vi "Calibrate LCVR_Capture.vi"(8 "error in (no error)":errorcluster {"code" format="%.0x"}, 10 "Handle in":u32, 11 "Buffer Info":T1) -> (0 "error out":errorcluster, 1 "Image":dbl[][](graph), 2 "Handle out":u32, 3 "contrast":dbl)   [LabVIEW 2012]
panel:
  out "frame":i32
  out "Frame Count":i32
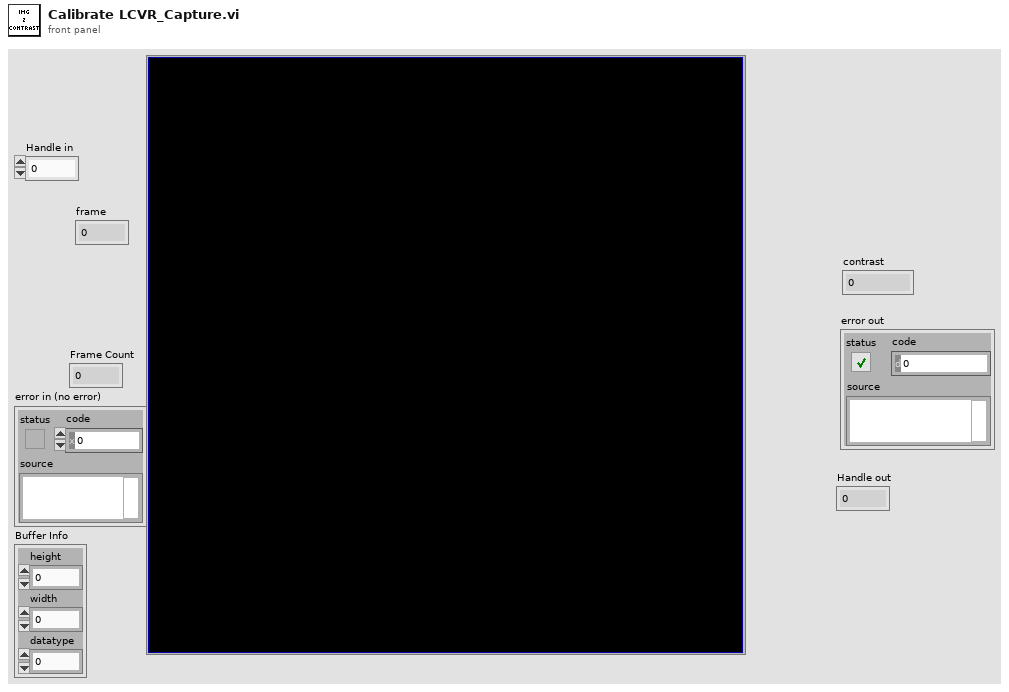
[diagram p1: front panel]
types:
  T1 = cluster{"height":u32, "width":u32, "datatype":u32}
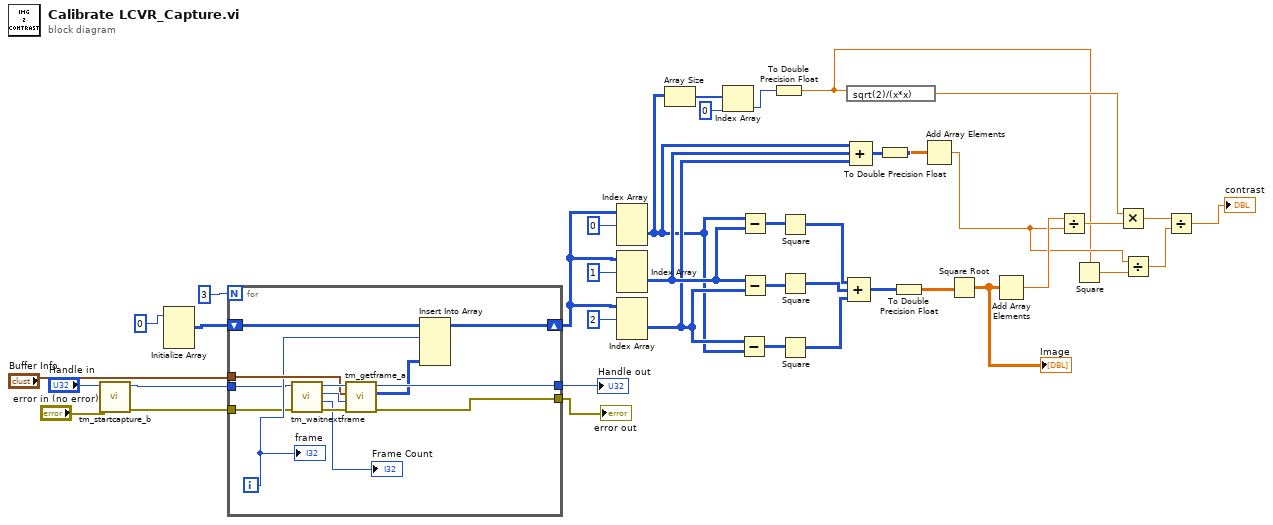
[diagram p0: block diagram]
diagram:
  n1 = call <userlib>:"tm_startcapture_b.vi"("error in (no error)"="error in (no error)", "Handle in"="Handle in") -> ("error out"=w36:errorcluster, "Handle out"=w37:u32)  [unwired: 8 in]
  n2 = Initialize Array(u16 0 ("element")) -> (w39:u16[][][])  [unwired: 3 in]
  n3 = for {
    N: 3 -> [_]
    tunnel: "Buffer Info" -> [w50]
    tunnel: [w49] -> w32
    tunnel: [w48] -> w31
    shift-right: [w46] -> w30
    shift-left: w39 -> [w47]
    tunnel: w37 -> [w43]
    tunnel: w36 -> [w42]
    i -> [w45]
    n4 = call <userlib>:"tm_waitnextframe.vi"("error in (no error)"=w42, "Handle in"=w43) -> ("error out"=w51:errorcluster, "Frame Count"=→"Frame Count":i32, "Frame Index"=w53:i32, "Handle out"=w52:u32)  [unwired: 6 in]
    n5 = call <userlib>:"tm_getframe_a.vi"("error in (no error)"=w51, "Frame Index"=w53, "Buffer Info"=w50, "Handle in"=w52) -> ("error out"=w48:errorcluster, "Data 16"=w41:u16[][], "Handle out"=w49:u32)  [unwired: 3 in, 2 out]
    n6 = Insert Into Array(array=w47, index (dim 0)=w45, new element=w41) -> (w46:u16[][][])  [unwired: 2 in]
    "frame" <- w45
  }
  "Handle out" <- w32
  "error out" <- w31
  n7 = Index Array(array=w30, index (dim 0)=0 ("index (page)")) -> (element=w16:u16[][])  [unwired: 2 in]
  n8 = Index Array(array=w30, index (dim 0)=1 ("index (page)")) -> (element=w19:u16[][])  [unwired: 2 in]
  n9 = Index Array(array=w30, index (dim 0)=2 ("index (page)")) -> (element=w18:u16[][])  [unwired: 2 in]
  n10 = Array Size(array=w16) -> (size(s)=w15:i32[])
  n11 = Index Array(array=w15, index=0) -> (element=w10:i32)
  n12 = Subtract(x=w18, y=w16) -> (x-y=w24:u16[][])
  n13 = Subtract(x=w16, y=w19) -> (x-y=w26:u16[][])
  n14 = Subtract(x=w19, y=w18) -> (x-y=w25:u16[][])
  n15 = To Double Precision Float(number=w10) -> (double precision float=w2:dbl)
  n16 = Square(x=w26) -> (x^2=w22:u16[][])
  n17 = Square(x=w25) -> (x^2=w21:u16[][])
  n18 = Square(x=w24) -> (x^2=w20:u16[][])
  n19 = expression code="sqrt(2)/(x*x)"(w2) -> (w12:dbl)
  n20 = Compound Arithmetic op=ADD(w22, w21, w20) -> (w23:u16[][])
  n21 = Compound Arithmetic op=ADD(w16, w19, w18) -> (w17:u16[][])
  n22 = To Double Precision Float(number=w17) -> (double precision float=w8:dbl[][])
  n23 = To Double Precision Float(number=w23) -> (double precision float=w7:dbl[][])
  n24 = Add Array Elements(numeric array=w8) -> (sum=w3:dbl)
  n25 = Square Root(x=w7) -> (sqrt(x)=w9:dbl[][])
  "Image" <- w9
  n26 = Add Array Elements(numeric array=w9) -> (sum=w13:dbl)
  n27 = Divide(x=w13, y=w3) -> (x/y=w11:dbl)
  n28 = Square(x=w2) -> (x^2=w1:dbl)
  n29 = Multiply(x=w12, y=w11) -> (x*y=w6:dbl)
  n30 = Divide(x=w3, y=w1) -> (x/y=w5:dbl)
  n31 = Divide(x=w6, y=w5) -> (x/y=→"contrast":dbl)
